vi "Check Number of Sessions.vi"(7 "require single session":bool, 8 "error in":errorcluster, 11 "sessions in":variant[](array[variant])) -> (0 "error out":errorcluster, 3 "sessions out":variant[](array[variant]))   [LabVIEW 2020, in "NI Session Management V1 Client.lvlib" / "Session Reservation.lvclass"]
uses:
  Session Reservation.lvclass
  Measurements/Helpers/Error Strings Global Internal.vi
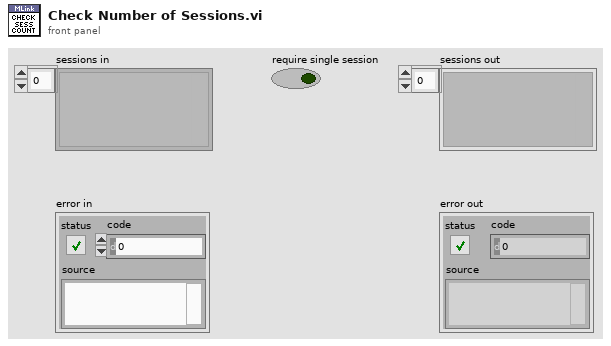
[diagram p1: front panel]
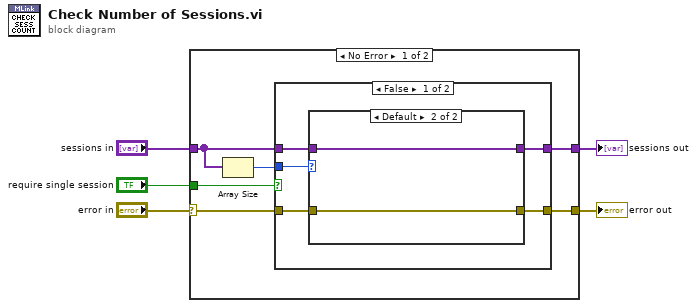
[diagram p0: block diagram]
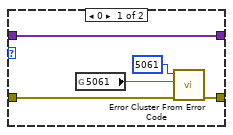
[diagram p2: hidden frame]
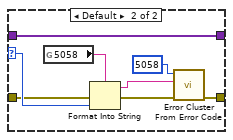
[diagram p4: hidden frame]
diagram:
  n1 = case shown="No Error" "error in" {
    selector: "error in" -> [w7 w39]
    tunnel: "sessions in" -> [w11 w40]
    tunnel: [w10 w40] -> w4
    tunnel: [w9 w39] -> w3
    tunnel: "require single session" -> [w8 _]
    frame No Error {
      n2 = Array Size(array=w11) -> (size(s)=w6:i32)
      n3 = case shown="False" w8 {
        tunnel: w11 -> [w16 w28]
        tunnel: [w15 w27] -> w10
        tunnel: [w13 w26] -> w9
        tunnel: w7 -> [w14 w25]
        tunnel: w6 -> [w12 w24]
        frame False {
          n4 = case shown="Default" w12 {
            tunnel: [w20 w23] -> w13
            tunnel: w16 -> [w17 w22]
            tunnel: w14 -> [w18 w23]
            tunnel: [w17 w22] -> w15
            frame 0 {
              n5 = global read "Error Strings Global Internal.vi" "5061"() -> (w19:string)
              n6 = call <vilib>:"Error Cluster From Error Code.vi"("error in (no error)"=w18, "error message (\"\")"=w19, "error code (0)"=5061) -> ("error out"=w20:errorcluster)  [unwired: 6 in]
            }
            frame Default {
            }
          }
        }
        frame True {
          n7 = case shown="1" w24 {
            selector: w24 -> [_ w36]
            tunnel: [w30 w37] -> w26
            tunnel: w28 -> [w29 w31]
            tunnel: w25 -> [w30 w34]
            tunnel: [w29 w31] -> w27
            frame 1 {
            }
            frame Default {
              n8 = global read "Error Strings Global Internal.vi" "5058"() -> (w35:string)
              n9 = Format Into String(format string=w35, error in=w34, w36) -> (resulting string=w32:string, error out=w33:errorcluster)  [unwired: 1 in]
              n10 = call <vilib>:"Error Cluster From Error Code.vi"("error in (no error)"=w33, "error message (\"\")"=w32, "error code (0)"=5058) -> ("error out"=w37:errorcluster)  [unwired: 6 in]
            }
          }
        }
      }
    }
    frame Error {
    }
  }
  "sessions out" <- w4
  "error out" <- w3
